vi "Acnet REST Multi-Device Reader.vi"(8 "error in (no error)":errorcluster, 10 "Devices":string[](array[string]), 11 "client handle":T1) -> (0 "error out":errorcluster, 2 "ACNET Device Readings":T2(array[cluster]), 3 "client handle out":T1)   [LabVIEW 2013]
uses:
  <vilib>/httpClient/ClientHandle.ctl
  <vilib>/httpClient/LabVIEWHTTPClient.lvlib
panel:
  out "expanded url":string
  out "headers":string
  out "body":string
  in  "url":string="http://www-bd.fnal.gov/getdaq/job/$(DEVICE_LIST)?type=xml&iso-time=true&quiet=true"
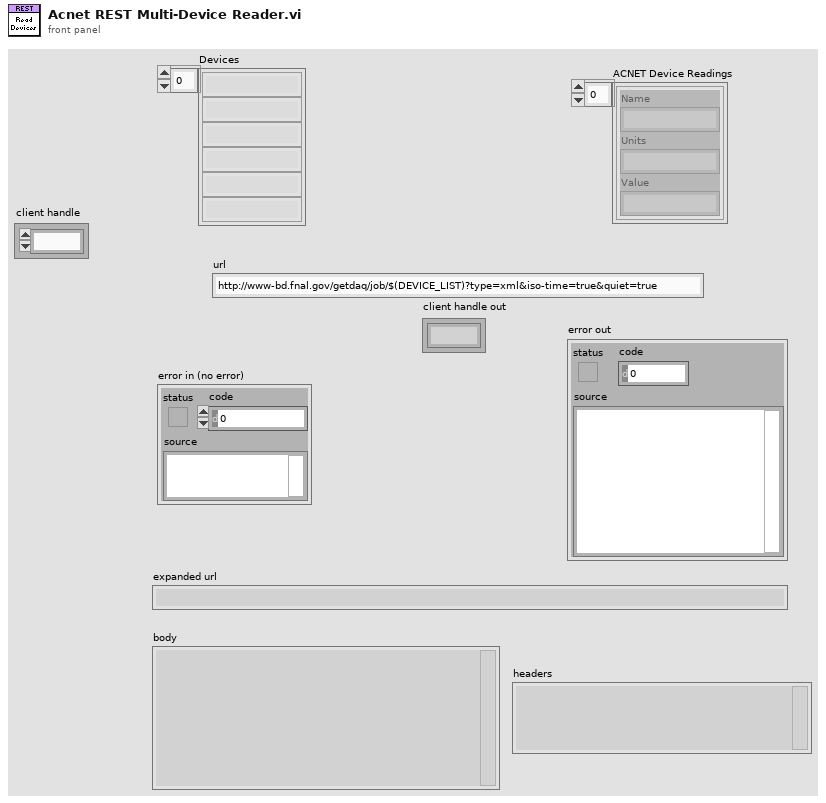
[diagram p1: front panel]
types:
  T1 = typedef "LabVIEWHTTPClient.lvlib/ClientHandle.ctl" = refnum<k1>
  T2 = cluster{"Name":string, "Units":string, "Value":string}[]
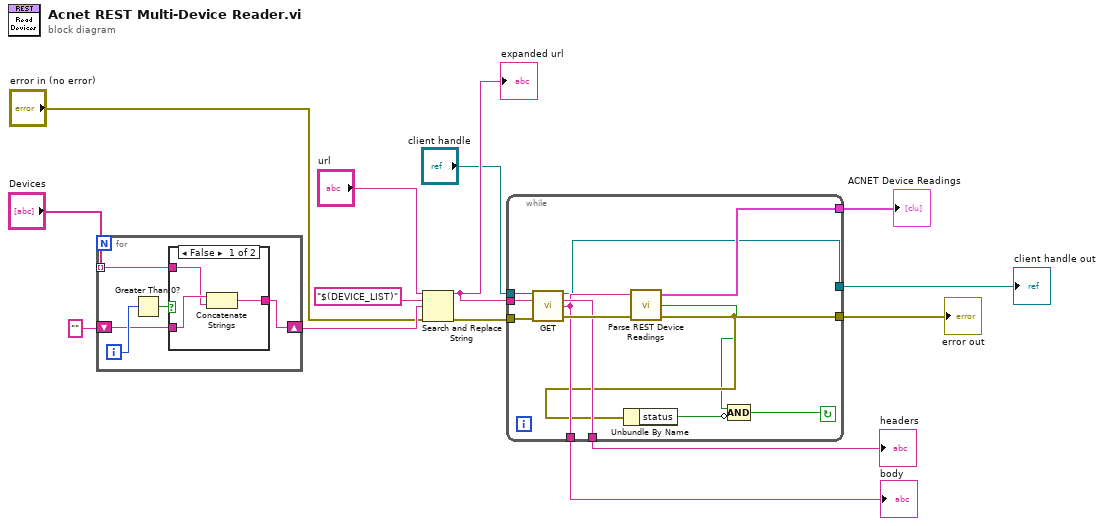
[diagram p0: block diagram]
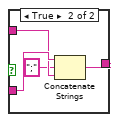
[diagram p2: hidden frame]
diagram:
  n1 = for {
    tunnel: "Devices" -> [w17] mode=indexing
    shift-right: [w15] -> w10
    shift-left: "" ("Device") -> [w16]
    i -> [w19]
    n2 = Greater Than 0?(x=w19) -> (x > 0?=w18:bool)
    n3 = case shown="False" w18 {
      tunnel: w17 -> [w21 w24]
      tunnel: w16 -> [w22 w26]
      tunnel: [w20 w25] -> w15
      frame False {
        n4 = Concatenate Strings(w22, w21) -> (w20:string)
      }
      frame True {
        n5 = Concatenate Strings(w26, ";" ("string"), w24) -> (w25:string)
      }
    }
  }
  n6 = Search and Replace String(input string="url", search string="$(DEVICE_LIST)", replace string=w10, error in="error in (no error)") -> (result string=w8:string, error out=w5:errorcluster)  [unwired: 4 in, 2 out]
  "expanded url" <- w8
  n7 = while {
    tunnel: w5 -> [w38]
    tunnel: [w32] -> w4
    tunnel: w8 -> [w37]
    tunnel: [w35] -> w7
    tunnel: [w34] -> w6
    tunnel: [w33] -> w3
    tunnel: "client handle" -> [w28]
    tunnel: [w27] -> w2
    stop <- w31 continue-if-true
    n8 = call <vilib>:"GET.vi"("client handle"=w28, "url"=w37, "error in (no error)"=w38) -> ("client handle out"=w27:T1, "headers"=w35:string, "body"=w34:string, "error out"=w36:errorcluster)  [unwired: 9 in]
    n9 = call "Parse REST Device Readings.vi"("error in (no error)"=w36, "Reading XML"=w34) -> ("error out"=w32:errorcluster, "Pending"=w29:bool, "ACNET Device Readings"=w33:T2)  [unwired: 1 in]
    n10 = Unbundle By Name(w32) -> ("status"=w30:bool)
    n11 = Compound Arithmetic op=AND(w29, invert w30) -> (w31:bool)
  }
  "error out" <- w4
  "headers" <- w7
  "body" <- w6
  "ACNET Device Readings" <- w3
  "client handle out" <- w2
